vi "搜索.vi"() -> ()   [LabVIEW 2017]
uses:
  <vilib>/Utility/miscctls.llb/LVRowAndColumnUnsignedTypeDef.ctl
panel:
  in  "停止按钮":bool
  out "提示框":string
  in  "类层次结构":i32(listbox)
  in  "筛选结果":i32(listbox)
  in  "本地类名搜索":string
  # ">>"
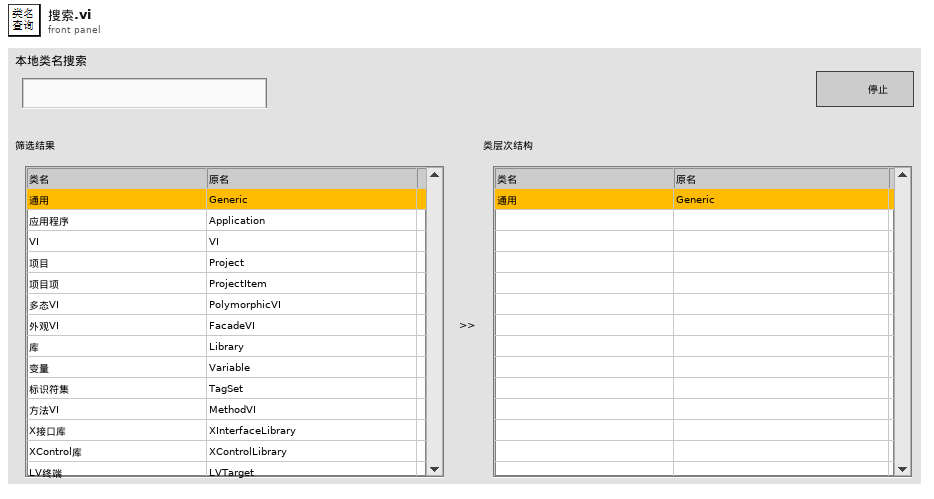
[diagram p1: front panel]
types:
  T1 = typedef "ASC_ArrayOfUniqueIDStringParentIDStringName.ctl" = T2[]
  T2 = typedef "ASC_UniqueIDStringParentIDStringName.ctl" = cluster{"Unique ID string":string, "Parent ID string":string, "Class Name (unlocalized)":string, "Class Name (localized)":string}
  T3 = typedef "LVRowAndColumnUnsignedTypeDef.ctl" = cluster{"Row":u32, "Column":u32}
  T4 = typedef "LVPoint32TypeDef.ctl" = cluster{"Horizontal":i32, "Vertical":i32}
  T5 = typedef "LVRowAndColumnTypeDef.ctl" = cluster{"Row":i32, "Column":i32}
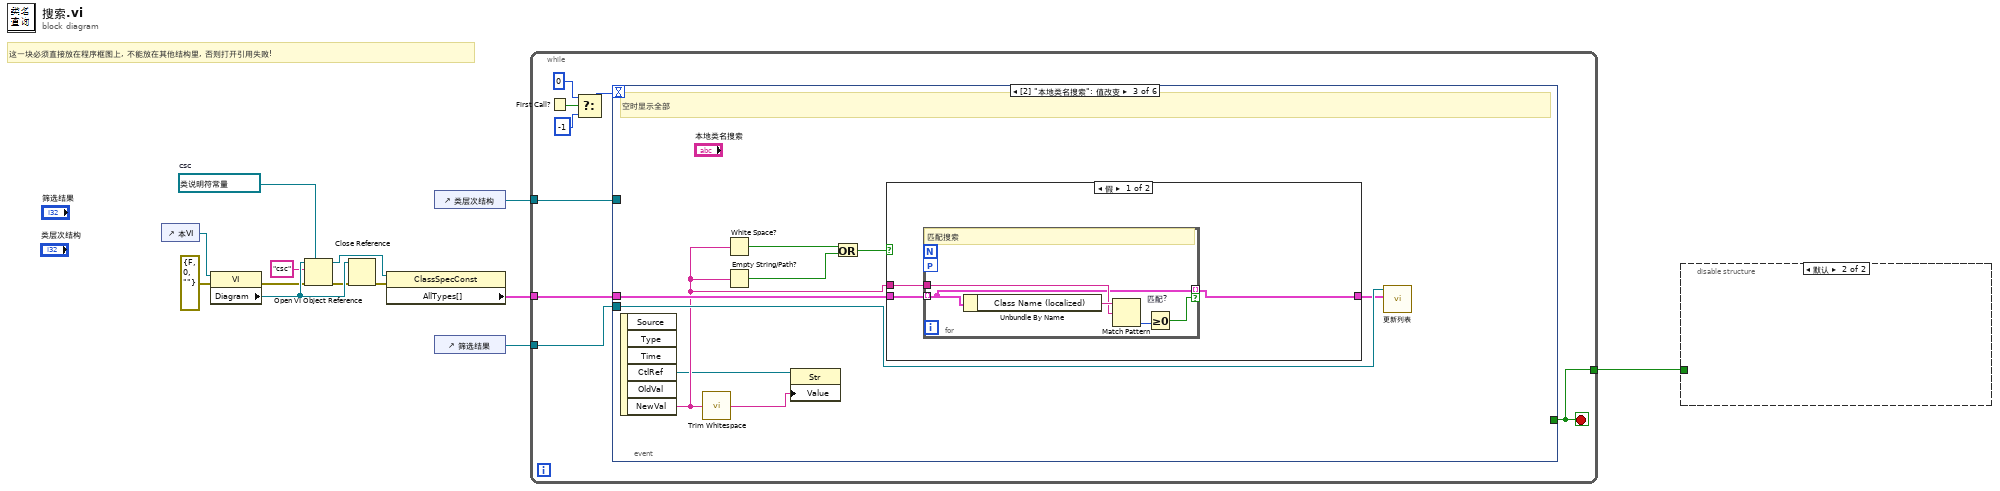
[diagram p0: block diagram]
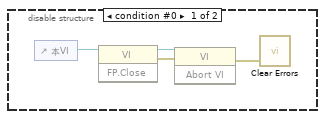
[diagram p2: hidden frame]
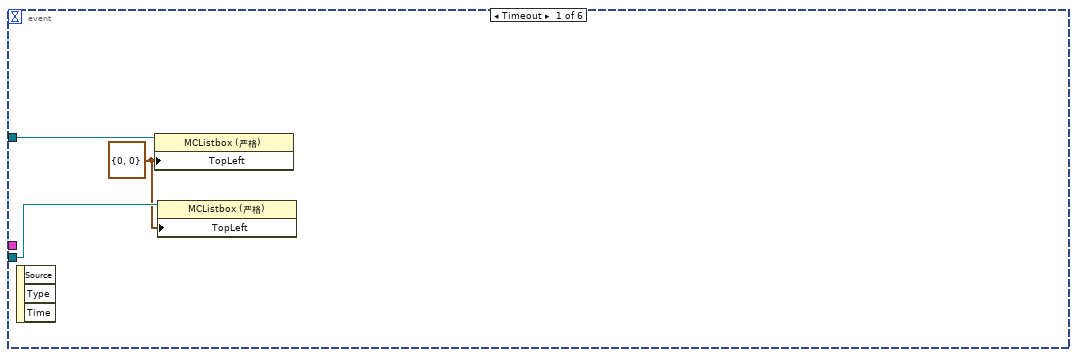
[diagram p3: hidden frame]
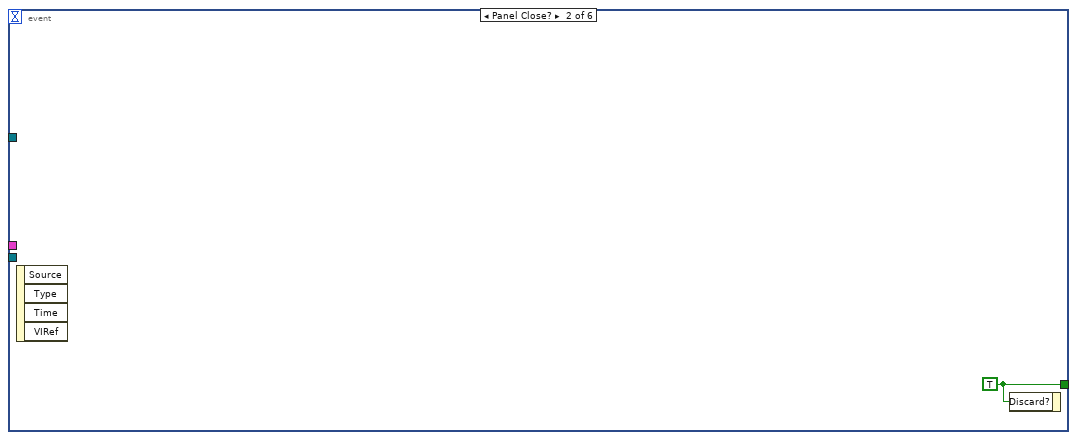
[diagram p4: hidden frame]
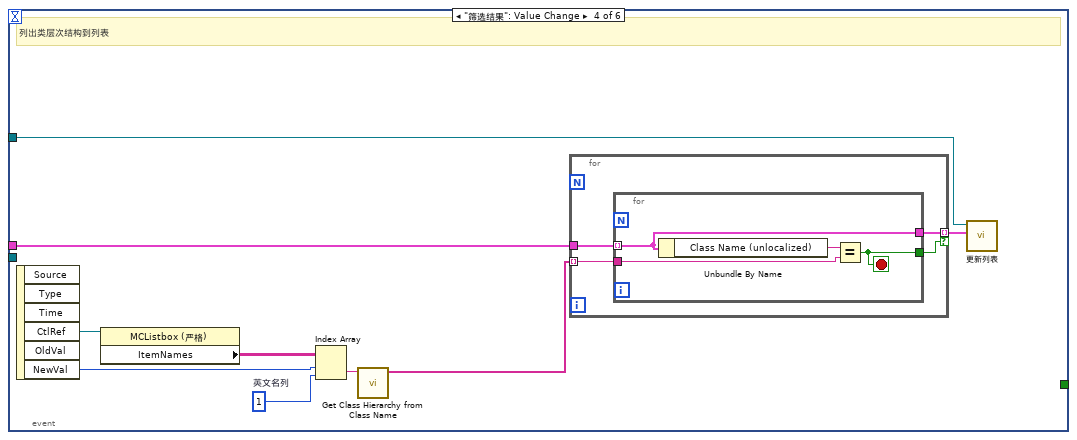
[diagram p6: hidden frame]
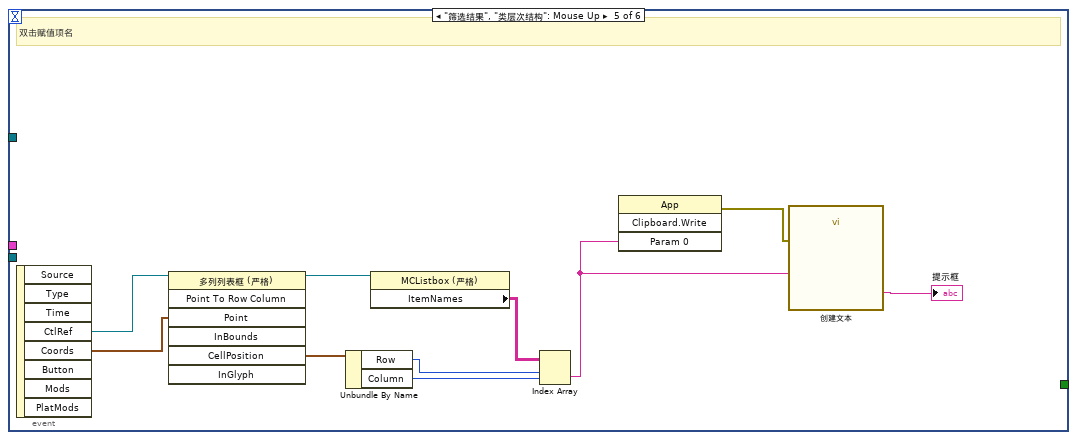
[diagram p7: hidden frame]
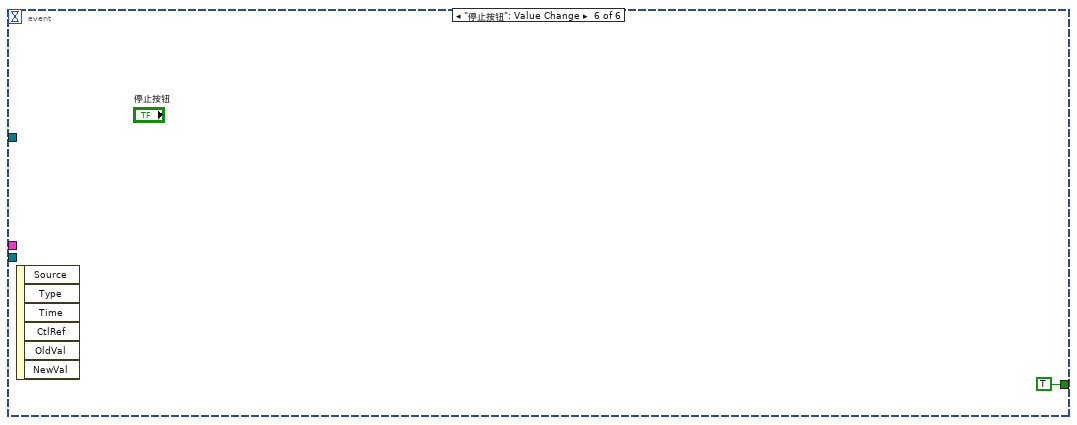
[diagram p8: hidden frame]
diagram:
  w3 = refnum<vi> refnum  # csc
  # "这一块必须直接放在程序框图上, 不能放在其他结构里, 否则打开引用失败!"
  n1 = control-ref of="本VI"() -> (w10:refnum<vi>)
  n2 = property class="VI"(reference=w10, error in=errorcluster {"status"=FALSE, "code"=0, "source"=""} ("错误输入（无错误）")) -> (error out=w5:errorcluster, "Diagram"=w8:refnum<vi>)  [unwired: 1 out]
  n3 = Open VI Object Reference(7:w3, 8:w5, 10:"csc" ("name/order"), 11:w8) -> (0:w6:errorcluster, 3:w9:refnum<vi>)
  n4 = Close Reference(reference=w8, error in (no error)=w6) -> (error out=w7:errorcluster)
  n5 = property class="ClassSpecConst"(reference=w9, error in=w7) -> ("AllTypes[]"=w11:T1)  [unwired: 2 out]
  n6 = control-ref of="类层次结构"() -> (w12:refnum<vi>)
  n7 = control-ref of="筛选结果"() -> (w13:refnum<vi>)
  n8 = while {
    tunnel: w11 -> [w21]
    tunnel: w13 -> [w20]
    tunnel: w12 -> [w19]
    tunnel: [w18] -> w1
    stop <- w18 stop-if-true
    n9 = First Call?() -> (First Call?: T/F=w17:bool)
    n10 = Select(t=0, s=w17, f=-1) -> (s? t:f=w16:i32)
    n11 = event shown="[2] \"本地类名搜索\": 值改变" {
      selector: _ -> [_ _ _ _ _ _]
      dyn-events: _ -> [_ _ _ _ _ _]
      timeout: w16 -> [_ _ _ _ _ _]
      tunnel: w21 -> [_ _ w31 w46 _ _]
      tunnel: w20 -> [w24 _ w30 _ _ _]
      tunnel: w19 -> [w23 _ _ w44 _ _]
      tunnel: [_ w25 _ _ _ TRUE ("放弃？")] -> w18
      event Timeout {
        w22 = T3 {"Row"=0, "Column"=0} ("左上可见单元格")
        n12 = event-data() -> ()  [unwired: 1 in, 3 out]
        n13 = property class="MCListbox (严格)"(reference=w23, "TopLeft"=w22) -> ()  [unwired: 1 in, 2 out]
        n14 = property class="MCListbox (严格)"(reference=w24, "TopLeft"=w22) -> ()  [unwired: 1 in, 2 out]
      }
      event Panel Close? {
        w25 = TRUE ("放弃？")
        n15 = event-data() -> ()  [unwired: 1 in, 4 out]
        n16 = event-data("Discard?"=w25) -> ()  [unwired: 1 in, 1 out]
      }
      event "本地类名搜索": Value Change {
        # "空时显示全部"
        n17 = event-data() -> ("CtlRef"=w26:refnum<vi>, "NewVal"=w28:string)  [unwired: 1 in, 4 out]
        n18 = call <vilib>:"Trim Whitespace.vi"("string"=w28) -> ("trimmed string"=w27:string)  [unwired: 1 in]
        n19 = White Space?(1:w28) -> (0:w34:bool)
        n20 = Empty String/Path?(string/path=w28) -> (empty?=w33:bool)
        n21 = property class="Str"(reference=w26, "Value"=w27) -> ()  [unwired: 1 in, 2 out]
        n22 = Or(x=w34, y=w33) -> (x .or. y?=w32:bool)
        n23 = case shown="假" w32 {
          tunnel: w31 -> [w37 w43]
          tunnel: w28 -> [w36 _]
          tunnel: [w35 w43] -> w29
          frame False {
            n24 = for {
              tunnel: [w38] -> w35 mode=indexing if=w39
              tunnel: w36 -> [w41]
              tunnel: w37 -> [w38] mode=indexing
              workers-P: _ -> [_]
              # "匹配搜索"
              n25 = Unbundle By Name(w38) -> ("Class Name (localized)"=w42:string)
              n26 = Match Pattern(string=w42, regular expression=w41) -> (offset past match=w40:i32)  [unwired: 1 in, 3 out]
              n27 = Greater Or Equal To 0? "匹配?"(x=w40) -> (x >= 0?=w39:bool)
            }
          }
          frame True {
            # "空 或 空白 ,则显示全部"
          }
        }
        n28 = call "更新列表.vi"("VI Server Class Info Array"=w29, "列表框引用 i"=w30) -> ()  [unwired: 9 in, 1 out]
      }
      event "筛选结果": Value Change {
        w49 = 1  # 英文名列
        # "列出类层次结构到列表"
        n29 = event-data() -> ("CtlRef"=w52:refnum<vi>, "NewVal"=w50:i32)  [unwired: 1 in, 4 out]
        n30 = property class="MCListbox (严格)"(reference=w52) -> ("ItemNames"=w51:string[][])  [unwired: 1 in, 2 out]
        n31 = Index Array(array=w51, index (row)=w50, index (col)=w49) -> (element=w48:string)
        n32 = call <vilib>:"Get Class Hierarchy from Class Name.vi"("Class Name"=w48) -> ("Class Hierarchy"=w47:string[])  [unwired: 9 in, 1 out]
        n33 = for {
          tunnel: w47 -> [w55] mode=indexing
          tunnel: w46 -> [w56]
          tunnel: [w54] -> w45 mode=indexing if=w53
          n34 = for {
            tunnel: w56 -> [w58] mode=indexing
            tunnel: w55 -> [w60]
            tunnel: [w58] -> w54
            tunnel: [w57] -> w53
            stop <- w57 stop-if-true
            n35 = Unbundle By Name(w58) -> ("Class Name (unlocalized)"=w59:string)
            n36 = Equal?(x=w59, y=w60) -> (x = y?=w57:bool)
          }
        }
        n37 = call "更新列表.vi"("VI Server Class Info Array"=w45, "列表框引用 i"=w44) -> ()  [unwired: 9 in, 1 out]
      }
      event "筛选结果", "类层次结构": Mouse Up {
        # "双击赋值项名"
        n38 = event-data() -> ("CtlRef"=w70:refnum<vi>, "Coords"=w69:T4)  [unwired: 1 in, 6 out]
        n39 = invoke class="多列列表框 (严格)" method="Point To Row Column"(reference=w70, "Point"=w69) -> (reference out=w68:refnum<vi>, "CellPosition"=w66:T5)  [unwired: 5 in, 5 out]
        n40 = Unbundle By Name(w66) -> ("Row"=w65:i32, "Column"=w64:i32)
        n41 = property class="MCListbox (严格)"(reference=w68) -> ("ItemNames"=w67:string[][])  [unwired: 1 in, 2 out]
        n42 = Index Array(array=w67, index (row)=w65, index (col)=w64) -> (element=w62:string)
        n43 = invoke class="App" method="Clipboard.Write"("Param 0"=w62) -> (error out=w61:errorcluster)  [unwired: 3 in, 3 out]
        n44 = call "创建文本"("复制项"=w62, "error in (no error)"=w61) -> ("Result"=→"提示框":string)  [unwired: 12 in, 1 out]
      }
      event "停止按钮": Value Change {
        n45 = event-data() -> ()  [unwired: 1 in, 6 out]
      }
    }
  }
  n46 = disable-structure shown="默认" {
    disable-tunnel: w1 -> [_ _]
    frame condition #0 {
      n47 = control-ref of="本VI"() -> (w72:refnum<vi>)
      n48 = invoke class="VI" method="FP.Close"(reference=w72) -> (reference out=w73:refnum<vi>, error out=w74:errorcluster)  [unwired: 2 in, 1 out]
      n49 = invoke class="VI" method="Abort VI"(reference=w73, error in=w74) -> (error out=w75:errorcluster)  [unwired: 1 in, 2 out]
      n50 = call <vilib>:"Clear Errors.vi"("error in (no error)"=w75) -> ()  [unwired: 5 in, 2 out]
    }
    frame condition #1 (active) {
    }
  }
